vi "Set Database Item Type.vi"(8 "error in (no error)":errorcluster, 9 "type id":u32, 10 "database item id":u32, 11 "eLab in":refnum<class "PL eLabFTW Client.lvclass">) -> (0 "error out":errorcluster, 3 "eLab out":refnum<class "PL eLabFTW Client.lvclass">)   [LabVIEW 2015, in "PL eLabFTW Client.lvclass"]
doc: "Sets database item type."
uses:
  PL eLabFTW Client.lvclass
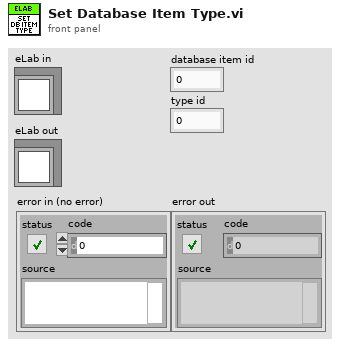
[diagram p1: front panel]
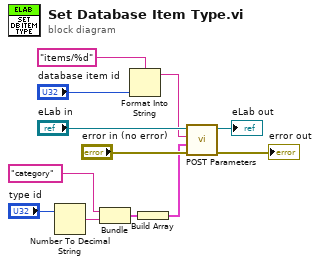
[diagram p0: block diagram]
diagram:
  n1 = Number To Decimal String(number="type id") -> (decimal integer string=w3:string)  [unwired: 1 in]
  n2 = Bundle("format string"="category", w3) -> (w5:cluster{"format string":string, string})  [unwired: 1 in]
  n3 = Format Into String(format string="items/%d", "database item id") -> (resulting string=w6:string)  [unwired: 2 in, 1 out]
  n4 = Build Array(w5) -> (w1:cluster{"format string":string, string}[])
  n5 = call "POST Parameters.vi"("error in (no error)"="error in (no error)", "parameters"=w1, "relative URL"=w6, "eLab in"="eLab in") -> ("error out"=→"error out":errorcluster, "eLab out"=→"eLab out":refnum<class "PL eLabFTW Client.lvclass">)  [unwired: 5 in, 1 out]
